vi "Unflatten LIDAR Data.vi"(11 "Flat LIDAR Data":dbl[](array[numeric])) -> (0 "Robot Pose x,y (m)":dbl[](array[numeric]), 1 "Robot Pose Theta (rad)":dbl, 2 "Bearing (rad)":dbl[](array[numeric]), 3 "Range (m)":dbl[](array[numeric]))   [LabVIEW 2018]
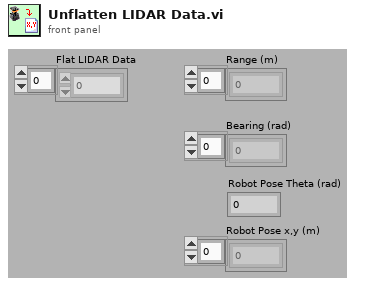
[diagram p1: front panel]
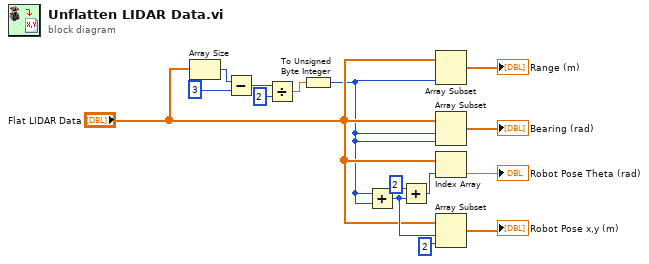
[diagram p0: block diagram]
diagram:
  n1 = Array Size(array="Flat LIDAR Data") -> (size(s)=w5:i32)
  n2 = Subtract(x=w5, y=3) -> (x-y=w4:i32)
  n3 = Divide(x=w4, y=2) -> (x/y=w2:dbl)
  n4 = To Unsigned Byte Integer(number=w2) -> (unsigned 8bit integer=w1:u8)
  n5 = Add(x=w1, y=w1) -> (x+y=w12:u8)
  n6 = Add(x=2 ("y"), y=w12) -> (x+y=w10:i32)
  n7 = Array Subset(array="Flat LIDAR Data", length=w1) -> (→"Range (m)":dbl[])  [unwired: 1 in]
  n8 = Array Subset(array="Flat LIDAR Data", index=w1, length=w1) -> (→"Bearing (rad)":dbl[])
  n9 = Index Array(array="Flat LIDAR Data", index=w10) -> (element=→"Robot Pose Theta (rad)":dbl)
  n10 = Array Subset(array="Flat LIDAR Data", index=w12, length=2) -> (→"Robot Pose x,y (m)":dbl[])
